vi "Cubed.vi"(10 "X":dbl) -> (2 "X^3":dbl)   [LabVIEW 2019]
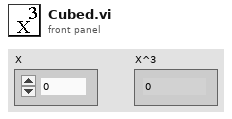
[diagram p1: front panel]
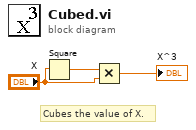
[diagram p0: block diagram]
diagram:
  # "Cubes the value of X."
  n1 = Square(x="X") -> (x^2=w3:dbl)
  n2 = Multiply(x=w3, y="X") -> (x*y=→"X^3":dbl)
